vi "Config Frequency.vi"(0 "VISA Resource Name":refnum<visa-resource-name>, 1 "Freq Offset (0.0)":dbl format="%#_3g", 2 "Freq Multiplier (1.0)":dbl=1.0, 3 "Adjust Phase (0.0)":dbl format="%.3f", 5 "Frequency (1000.0)":dbl=1000.0 format="%#.3g", 7 "Freq Ref Set (0.0)":dbl format="%.8f", 9 "Freq Ref (T:ON)":bool=TRUE, 11 "error in (no error)":errorcluster {"code" format="%.0x"}, 12 "OptPhNoise (F:MD2 > 10khzOffset)":bool) -> (4 "VISA Resource Name Out":refnum<visa-resource-name>, 15 "error out":errorcluster {"code" format="%.0x"})   [LabVIEW 2014, in "Agilent ESG Series.lvlib"]
doc: "This VI is used to set the modulation controls and the parameters associated with the carrier signal frequency.\n\nNotes:\nThis VI is used with ESG-A and ESG-D Series instruments only."
uses:
  Agilent ESG Series.lvlib
panel:
  # "MODE 1 < 10khz Offset"
  # "MODE 2 >10khz Offset"
  # "ON"
  # "OFF"
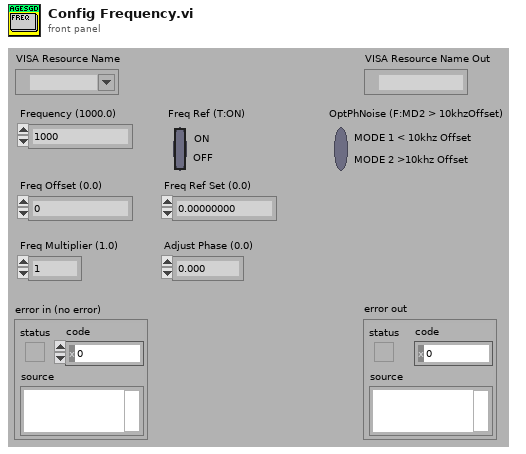
[diagram p1: front panel]
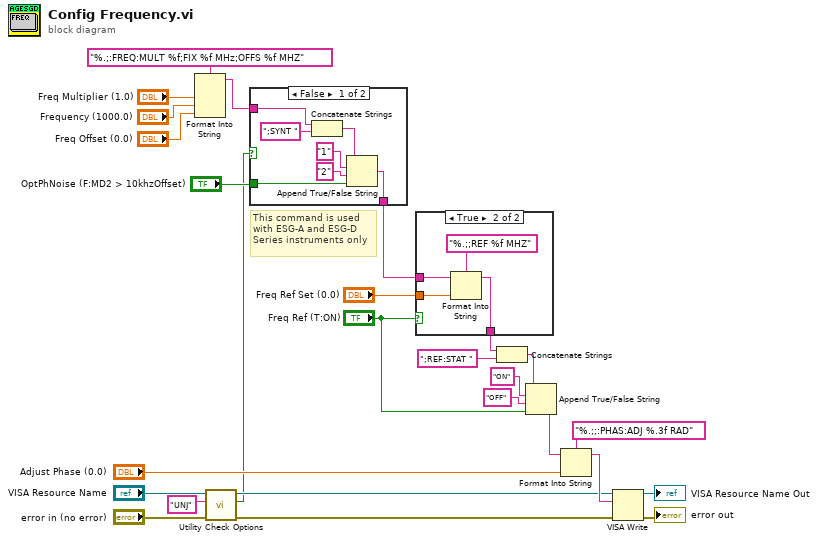
[diagram p0: block diagram]
diagram:
  # "This command is used \nwith ESG-A and ESG-D \nSeries instruments only"
  n1 = Format Into String(format string="%.;:FREQ:MULT %f;FIX %f MHz;OFFS %f MHZ", "Freq Multiplier (1.0)", "Frequency (1000.0)", "Freq Offset (0.0)") -> (resulting string=w7:string)  [unwired: 2 in, 1 out]
  n2 = call "Utility Check Options.vi"("error in (no error)"="error in (no error)", "Search Options"="UNJ", "VISA Resource Name"="VISA Resource Name") -> ("error out"=w12:errorcluster, "Found"=w3:bool, "VISA Resource Name Out"=w14:refnum<visa-resource-name>)  [unwired: 6 in]
  n3 = case shown="False" w3 {
    tunnel: w7 -> [w29 w34]
    tunnel: "OptPhNoise (F:MD2 > 10khzOffset)" -> [w28 _]
    tunnel: [w27 w34] -> w6
    frame False {
      n4 = Concatenate Strings(w29, ";SYNT ") -> (w32:string)
      n5 = Append True/False String(1:w28, 2:"2" ("false string"), 3:"1" ("true string"), 4:w32) -> (0:w27:string)
    }
    frame True {
    }
  }
  n6 = case shown="True" "Freq Ref (T:ON)" {
    tunnel: [w35 w36] -> w5
    tunnel: "Freq Ref Set (0.0)" -> [_ w39]
    tunnel: w6 -> [w35 w37]
    frame False {
    }
    frame True {
      n7 = Format Into String(format string="%.;;REF %f MHZ", initial string=w37, w39) -> (resulting string=w36:string)  [unwired: 1 in, 1 out]
    }
  }
  n8 = Concatenate Strings(w5, ";REF:STAT ") -> (w23:string)
  n9 = Append True/False String(1:"Freq Ref (T:ON)", 2:"OFF" ("false string"), 3:"ON" ("true string"), 4:w23) -> (0:w1:string)
  n10 = Format Into String(format string="%.;;:PHAS:ADJ %.3f RAD", initial string=w1, "Adjust Phase (0.0)") -> (resulting string=w18:string)  [unwired: 1 in, 1 out]
  n11 = VISA Write(VISA resource name=w14, write buffer=w18, error in (no error)=w12) -> (VISA resource name out=→"VISA Resource Name Out":refnum<visa-resource-name>, error out=→"error out":errorcluster)  [unwired: 1 out]
